vi "Ramp_Bias_Modulation.vi"(0 "Sampling frequency (20000) / Hz":dbl=20000.0, 1 "Ramp Amplitude (1) / V":dbl=1.0, 2 "DC time (0.02) / s":dbl=0.02, 3 "Text Ring":u16(ring) items=["DC Bias", "square", "sine", "triangle", "IV", "IV - Polarity Sweep", "CV - 2 terminal", "Pre/Post Pulse IV"], 5 "DC Bias (0.2) / V":dbl=0.2, 9 "Ramp Length (0.1) / s":dbl=0.1, 11 "Error In":errorcluster, 12 "Pulse bias /V":dbl=2.0, 13 "Modulation Frequency (100) / Hz":dbl=100.0) -> (4 "Bias Ramp Out / V":dbl[](array[numeric]), 15 "Error Out":errorcluster)   [LabVIEW 2025]
uses:
  <vilib>/Analysis/NI_AALBase.lvlib
panel:
  out "Waveform Graph":dbl[](graph)
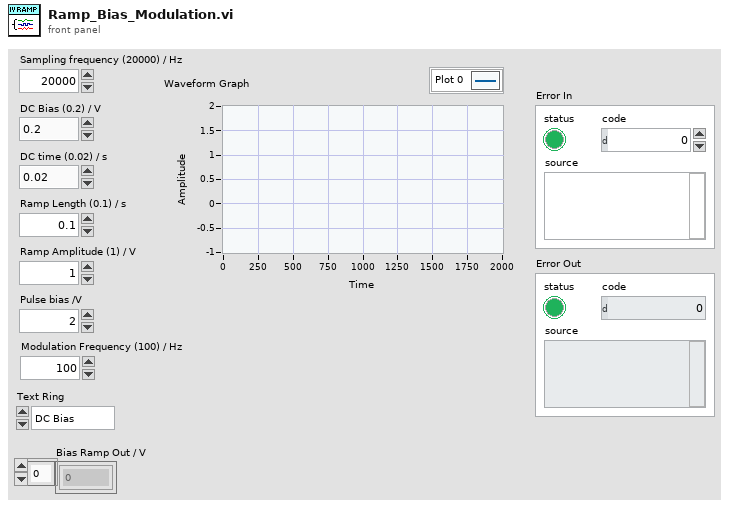
[diagram p1: front panel]
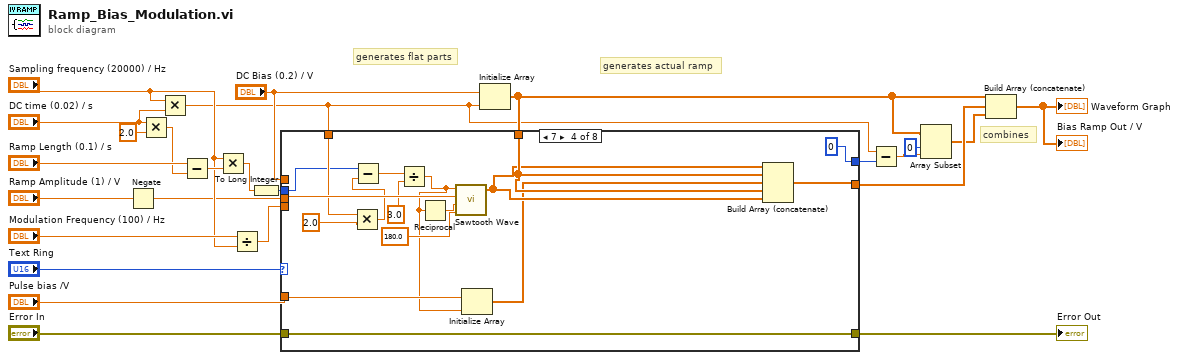
[diagram p0: block diagram]
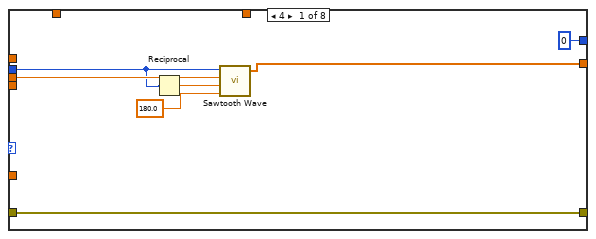
[diagram p2: hidden frame]
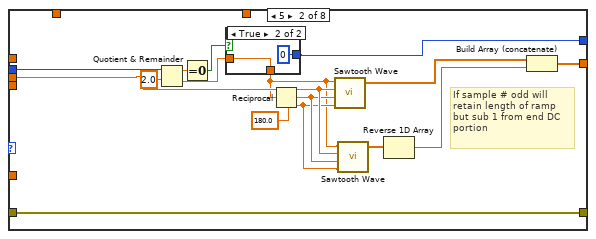
[diagram p3: hidden frame]
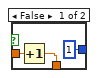
[diagram p4: hidden frame]
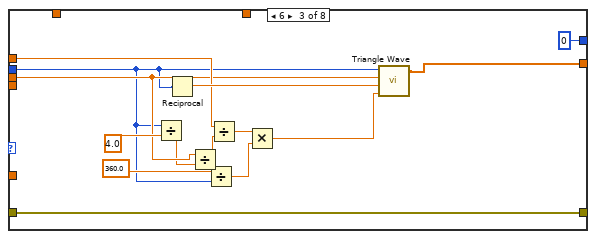
[diagram p5: hidden frame]
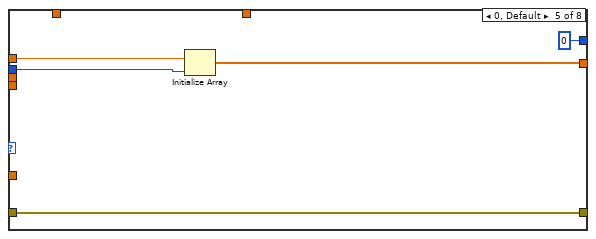
[diagram p6: hidden frame]
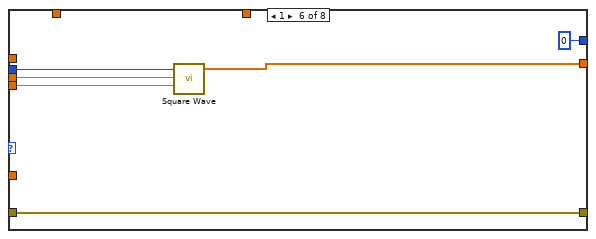
[diagram p7: hidden frame]
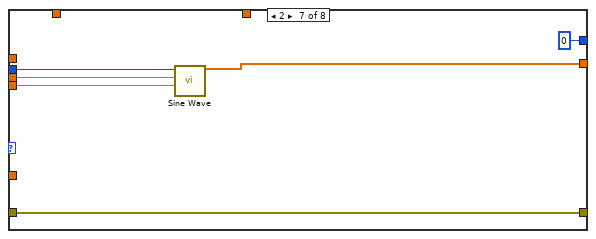
[diagram p8: hidden frame]
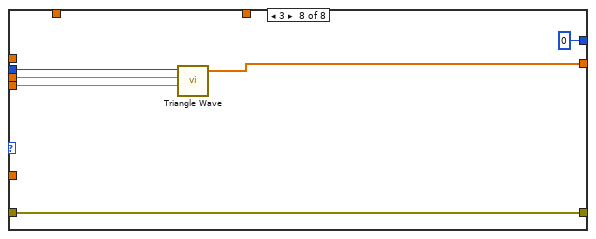
[diagram p9: hidden frame]
diagram:
  # "combines"
  # "generates actual ramp"
  # "generates flat parts"
  n1 = Negate(x="Ramp Amplitude (1) / V") -> (-x=w5:dbl)
  n2 = Multiply(x="DC time (0.02) / s", y=2.0) -> (x*y=w19:dbl)
  n3 = Multiply(x="Sampling frequency (20000) / Hz", y="DC time (0.02) / s") -> (x*y=w2:dbl)
  n4 = Subtract(x="Ramp Length (0.1) / s", y=w19) -> (x-y=w18:dbl)
  n5 = Multiply(x="Sampling frequency (20000) / Hz", y=w18) -> (x*y=w6:dbl)
  n6 = Divide(x="Modulation Frequency (100) / Hz", y="Sampling frequency (20000) / Hz") -> (x/y=w25:dbl)
  n7 = To Long Integer(number=w6) -> (32bit integer=w11:i32)
  n8 = Initialize Array("DC Bias (0.2) / V", w2) -> (w3:dbl[])
  n9 = case shown="7" "Text Ring" {
    tunnel: [w31 w47 w64 w68 w86 w90 w96 w102] -> w13
    tunnel: w5 -> [w32 w42 w55 w82 _ w93 w98 w106]
    tunnel: w11 -> [w27 w45 w53 w78 w88 w94 w99 w105]
    tunnel: w25 -> [_ _ _ _ _ w92 w97 w104]
    tunnel: "Error In" -> [w29 w43 w65 w67 w85 w91 w100 w103]
    tunnel: [w29 w43 w65 w67 w85 w91 w100 w103] -> w14
    tunnel: "DC Bias (0.2) / V" -> [_ _ w60 _ w87 _ _ _]
    tunnel: [0 w33 0 0 0 0 0 0] -> w10
    tunnel: w3 -> [_ _ _ w83 _ _ _ _]
    tunnel: w2 -> [_ _ _ w80 _ _ _ _]
    tunnel: "Pulse bias /V" -> [_ _ _ w72 _ _ _ _]
    frame 4 {
      n10 = Reciprocal(x=w27) -> (1/x=w28:dbl)
      n11 = call <vilib>:"Sawtooth Wave.vi"("samples"=w27, "amplitude"=w32, "frequency"=w28, "phase in"=180.0) -> ("sawtooth wave"=w31:dbl[])  [unwired: 1 in, 2 out]
    }
    frame 5 {
      w38 = 180.0 ("phase in")
      # "If sample # odd will\nretain length of ramp\nbut sub 1 from end DC\nportion"
      n12 = Quotient & Remainder(x=w45, y=2.0) -> (x-y*floor(x/y)=w44:dbl, floor(x/y)=w35:dbl)
      n13 = Equal To 0?(x=w44) -> (x = 0?=w36:bool)
      n14 = case shown="True" w36 {
        tunnel: w35 -> [w50 w52]
        tunnel: [w49 w52] -> w34
        tunnel: [1 0] -> w33
        frame False {
          n15 = Increment(x=w50) -> (x+1=w49:dbl)
        }
        frame True {
        }
      }
      n16 = Reciprocal(x=w34) -> (1/x=w39:dbl)
      n17 = call <vilib>:"Sawtooth Wave.vi"("samples"=w34, "amplitude"=w42, "frequency"=w39, "phase in"=w38) -> ("sawtooth wave"=w41:dbl[])  [unwired: 1 in, 2 out]
      n18 = call <vilib>:"Sawtooth Wave.vi"("samples"=w34, "amplitude"=w42, "frequency"=w39, "phase in"=w38) -> ("sawtooth wave"=w37:dbl[])  [unwired: 1 in, 2 out]
      n19 = Reverse 1D Array(array=w37) -> (reversed array=w40:dbl[])
      n20 = Build Array (concatenate)(w41, w40) -> (w47:dbl[])
    }
    frame 6 {
      n21 = Divide(x=w53, y=4.0) -> (x/y=w54:dbl)
      n22 = Reciprocal(x=w53) -> (1/x=w63:dbl)
      n23 = Divide(x=w55, y=w54) -> (x/y=w61:dbl)
      n24 = Divide(x=360.0, y=w53) -> (x/y=w58:dbl)
      n25 = Divide(x=w60, y=w61) -> (x/y=w59:dbl)
      n26 = Multiply(x=w59, y=w58) -> (x*y=w56:dbl)
      n27 = call <vilib>:"Triangle Wave.vi"("samples"=w53, "amplitude"=w55, "frequency"=w63, "phase in"=w56) -> ("triangle wave"=w64:dbl[])  [unwired: 1 in, 2 out]
    }
    frame 7 {
      n28 = Multiply(x=w80, y=2.0) -> (x*y=w79:dbl)
      n29 = Subtract(x=w78, y=w79) -> (x-y=w77:dbl)
      n30 = Divide(x=w77, y=3.0) -> (x/y=w71:dbl)
      n31 = Reciprocal(x=w71) -> (1/x=w75:dbl)
      n32 = call <vilib>:"Sawtooth Wave.vi"("samples"=w71, "amplitude"=w82, "frequency"=w75, "phase in"=180.0) -> ("sawtooth wave"=w73:dbl[])  [unwired: 1 in, 2 out]
      n33 = Initialize Array(w72, w71) -> (w70:dbl[])
      n34 = Build Array (concatenate)(w73, w83, w70, w83, w73) -> (w68:dbl[])
    }
    frame 0, Default {
      n35 = Initialize Array(w87, w88) -> (w86:dbl[])
    }
    frame 1 {
      n36 = call <vilib>:"Square Wave.vi"("samples"=w94, "amplitude"=w93, "frequency"=w92) -> ("square wave"=w90:dbl[])  [unwired: 3 in, 2 out]
    }
    frame 2 {
      n37 = call <vilib>:"Sine Wave.vi"("samples"=w99, "amplitude"=w98, "frequency"=w97) -> ("sine wave"=w96:dbl[])  [unwired: 2 in, 2 out]
    }
    frame 3 {
      n38 = call <vilib>:"Triangle Wave.vi"("samples"=w105, "amplitude"=w106, "frequency"=w104) -> ("triangle wave"=w102:dbl[])  [unwired: 2 in, 2 out]
    }
  }
  "Error Out" <- w14
  n39 = Subtract(x=w2, y=w10) -> (x-y=w9:dbl)
  n40 = Array Subset(array=w3, index=0, length=w9) -> (w7:dbl[])
  n41 = Build Array (concatenate)(w3, w13, w7) -> (→"Waveform Graph" →"Bias Ramp Out / V":dbl[])
